vi "Translator.vi"(0 "Input":variant, 11 "error in (no error)":errorcluster) -> (4 "Output":variant, 15 "error out":errorcluster)   [LabVIEW 2014, in "STM32F4 Discovery General Wrapper.lvlib"]
doc: "An example of how to create the Translator to convert the LabVIEW VIs to Arduino C code."
uses:
  <vilib>/Aledyne-TSXperts/Arduino Compatible Compiler for LabVIEW/addons/STM32F4 Discovery General Wrapper/STM32F4 Discovery General Wrapper.lvlib
panel:
  out "Outputs":string[](array[string])
  out "Inputs":string[](array[string])
  out "Output Datatypes":string[](array[string])
  out "Input Datatypes":string[](array[string])
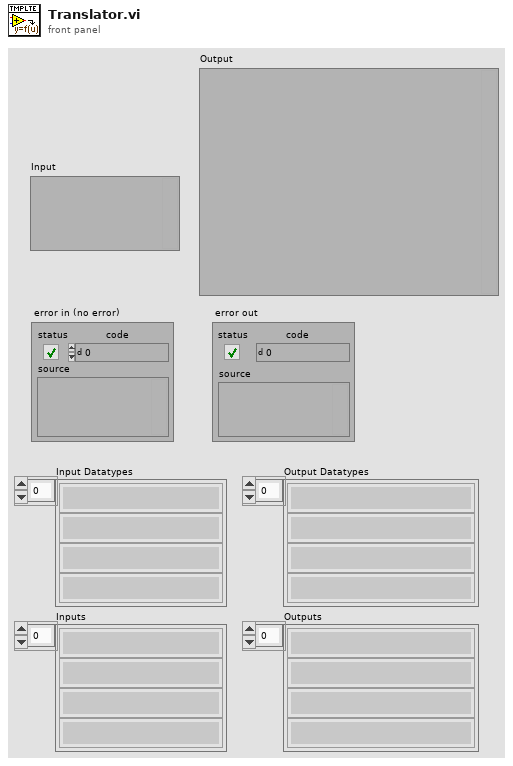
[diagram p1: front panel]
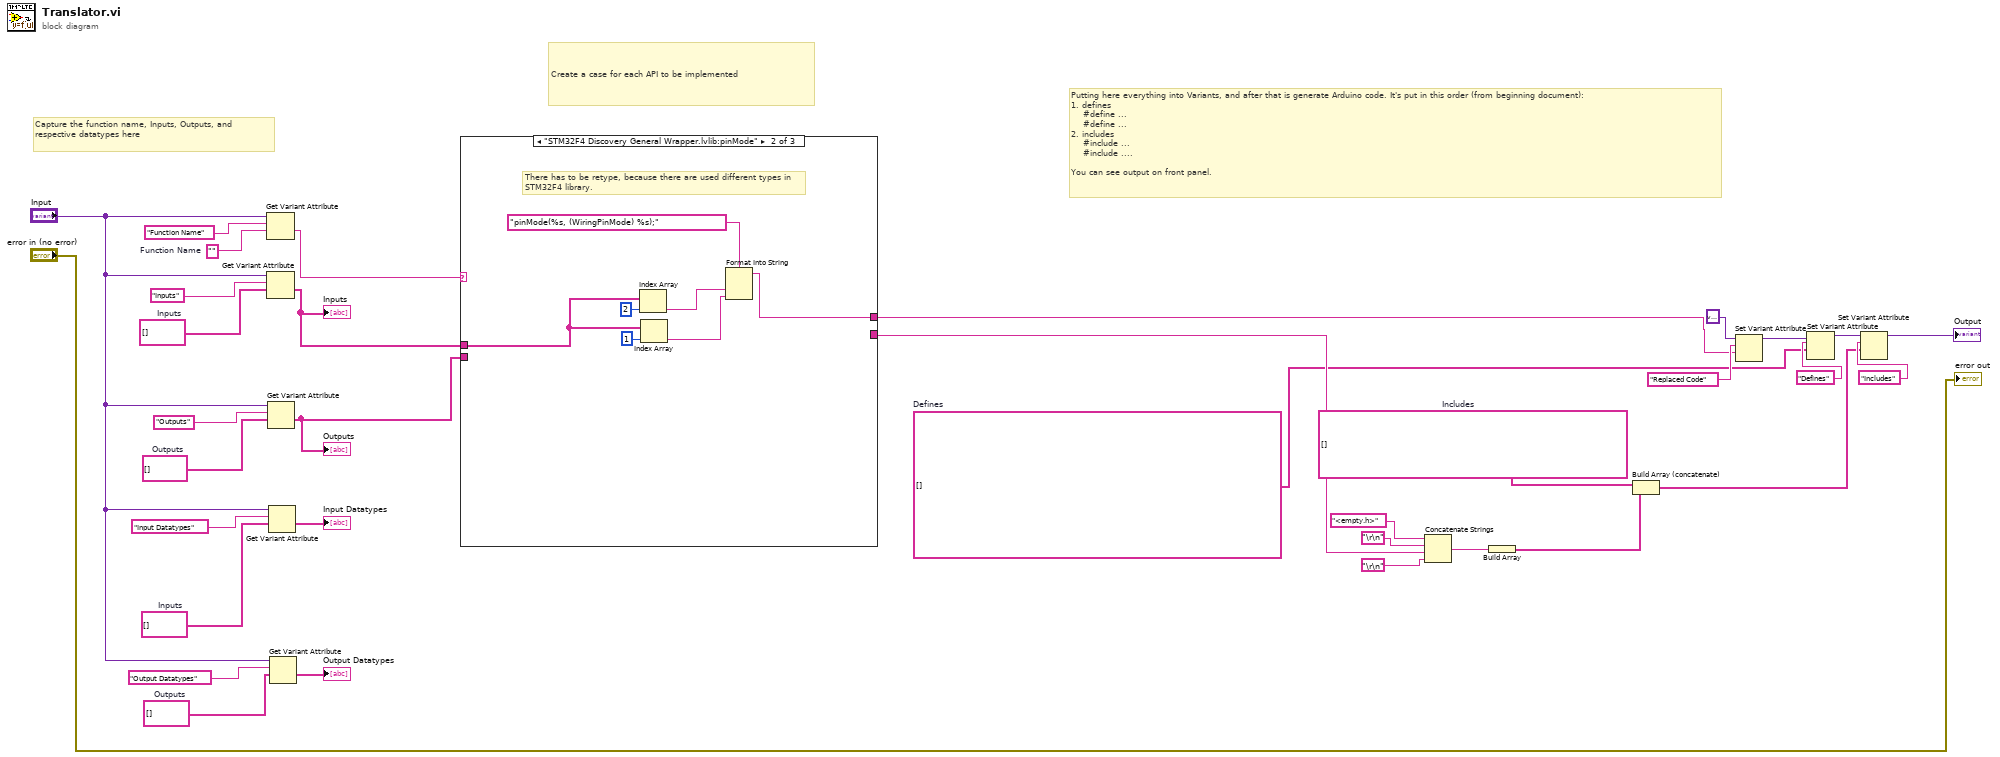
[diagram p0: block diagram]
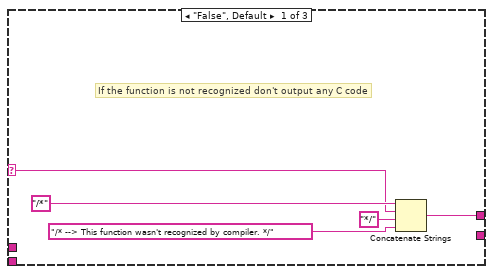
[diagram p2: hidden frame]
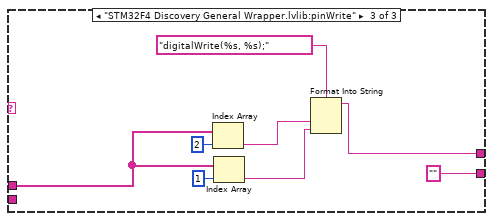
[diagram p3: hidden frame]
diagram:
  w1 = string[] []  # Defines
  w21 = string[] []  # Outputs
  w22 = string[] []  # Inputs
  w3 = string[] []  # Includes
  w30 = string[] []  # Outputs
  w31 = string[] []  # Inputs
  w32 = ""  # Function Name
  # "Capture the function name, Inputs, Outputs, and respective datatypes here"
  # "Putting here everything into Variants, and after that is generate Arduino code. It's put in this order (from beginning document):\n1. defines\n    #define ...\n    #define ...\n2. includes\n    #include ...\n    #include ....\n\nYou can see output on front panel."
  # "Create a case for each API to be implemented"
  n1 = Get Variant Attribute(Variant="Input", name="Function Name", default value (empty Variant)=w32) -> (value=w27:string)  [unwired: 1 in, 3 out]
  n2 = Get Variant Attribute(Variant="Input", name="Inputs", default value (empty Variant)=w31) -> (value=w17:string[])  [unwired: 1 in, 3 out]
  "Inputs" <- w17
  n3 = Get Variant Attribute(Variant="Input", name="Outputs", default value (empty Variant)=w30) -> (value=w18:string[])  [unwired: 1 in, 3 out]
  "Outputs" <- w18
  n4 = Get Variant Attribute(Variant="Input", name="Input Datatypes", default value (empty Variant)=w22) -> (value=→"Input Datatypes":string[])  [unwired: 1 in, 3 out]
  n5 = Get Variant Attribute(Variant="Input", name="Output Datatypes", default value (empty Variant)=w21) -> (value=→"Output Datatypes":string[])  [unwired: 1 in, 3 out]
  n6 = case shown="\"STM32F4 Discovery General Wrapper.lvlib:pinMode\"" w27 {
    selector: w27 -> [w37 _ _]
    tunnel: [w35 w40 w47] -> w26
    tunnel: w17 -> [_ w42 w49]
    tunnel: w18 -> [_ _ _]
    tunnel: [_ _ ""] -> w9
    frame "False", Default {
      # "If the function is not recognized don't output any C code"
      n7 = Concatenate Strings("/*" ("name"), w37, "*/" ("name"), "/* --> This function wasn't recognized by compiler. */" ("name")) -> (w35:string)
    }
    frame "STM32F4 Discovery General Wrapper.lvlib:pinMode" {
      # "There has to be retype, because there are used different types in\nSTM32F4 library."
      n8 = Index Array(array=w42, index=2) -> (element=w44:string)
      n9 = Index Array(array=w42, index=1) -> (element=w41:string)
      n10 = Format Into String(format string="pinMode(%s, (WiringPinMode) %s);", w44, w41) -> (resulting string=w40:string)  [unwired: 2 in, 1 out]
    }
    frame "STM32F4 Discovery General Wrapper.lvlib:pinWrite" {
      n11 = Index Array(array=w49, index=2) -> (element=w51:string)
      n12 = Index Array(array=w49, index=1) -> (element=w48:string)
      n13 = Format Into String(format string="digitalWrite(%s, %s);", w51, w48) -> (resulting string=w47:string)  [unwired: 2 in, 1 out]
    }
  }
  n14 = Concatenate Strings("<empty.h>" ("string"), "\r\n", w9, "\r\n") -> (w12:string)
  n15 = Build Array(w12) -> (w2:string[])
  n16 = Build Array (concatenate)(w3, w2) -> (w4:string[])
  n17 = Set Variant Attribute(Variant=variant ("variant"), name="Replaced Code", value=w26) -> (Variant out=w7:variant)  [unwired: 1 in, 2 out]
  n18 = Set Variant Attribute(Variant=w7, name="Defines", value=w1) -> (Variant out=w6:variant)  [unwired: 1 in, 2 out]
  n19 = Set Variant Attribute(Variant=w6, name="Includes", value=w4) -> (Variant out=→"Output":variant)  [unwired: 1 in, 2 out]
  "error out" <- "error in (no error)"
